vi "MDAQ_TestProgram.vi"() -> ()   [LabVIEW 2021]
uses:
  FunctionVIS/Status_Cluster.ctl
  FunctionVIS/CMD_ARG_Enum.ctl
  2434371f-5447-471b-b22c-6b5c2bc6bbb4.vi
panel:
  out "Delta4":dbl
  out "Delta 5":dbl
  out "Delta 3":dbl
  out "Delta 2":dbl
  out "Delta 1":dbl
  in  "stop":bool
  out "Intensity Graph":u32[][](graph)
  out "Test Ampl":T1(graph)
  in  "DeltaT":dbl
  in  "Freq":dbl
  in  "Bin":i32
  in  "VISA resource name":refnum<visa-resource-name>
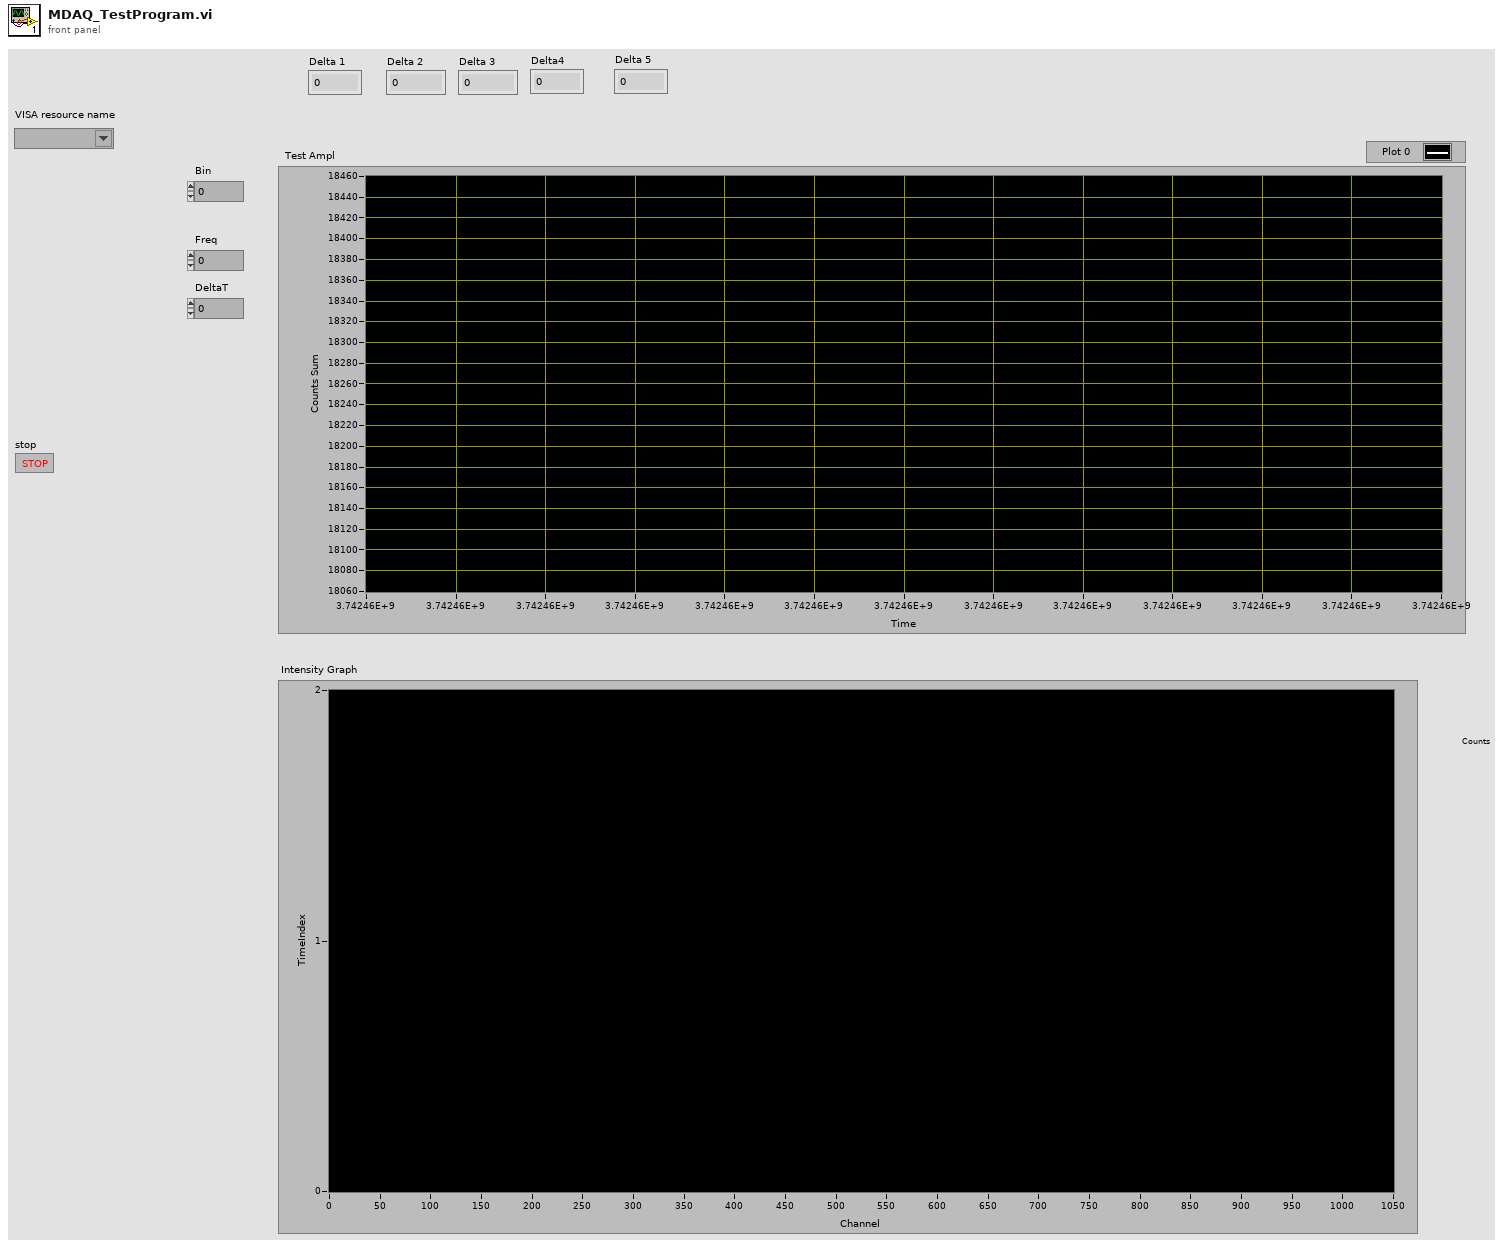
[diagram p1: front panel]
types:
  T1 = cluster{"seconds since 1Jan1904":timestamp, "sum":u32}[]
  T2 = typedef "Status_Cluster.ctl" = cluster{"CHAN":u32, "BASE":u32, "STEP":u32, "N_CYCLES":u32, "M_CYCLES":u32, "AMPLITUDE":u32, "GATESTRT":u32, "GATESTOP":u32, "Spectrum Array":u32[], "Spectrum Cycle":u32[][], "Cycle Timestamps":timestamp[], "Temperature Collect":dbl[]}
  T3 = typedef "CMD_ARG_Enum.ctl" = enum16{"N_Cycles", "GateStep", "ASCII_Spectrum", "Waveform", "GateStop", "GateStart", "Amplitude", "Frequency"}
  T4 = cluster{"seconds since 1Jan1904":timestamp, "sum":u32}
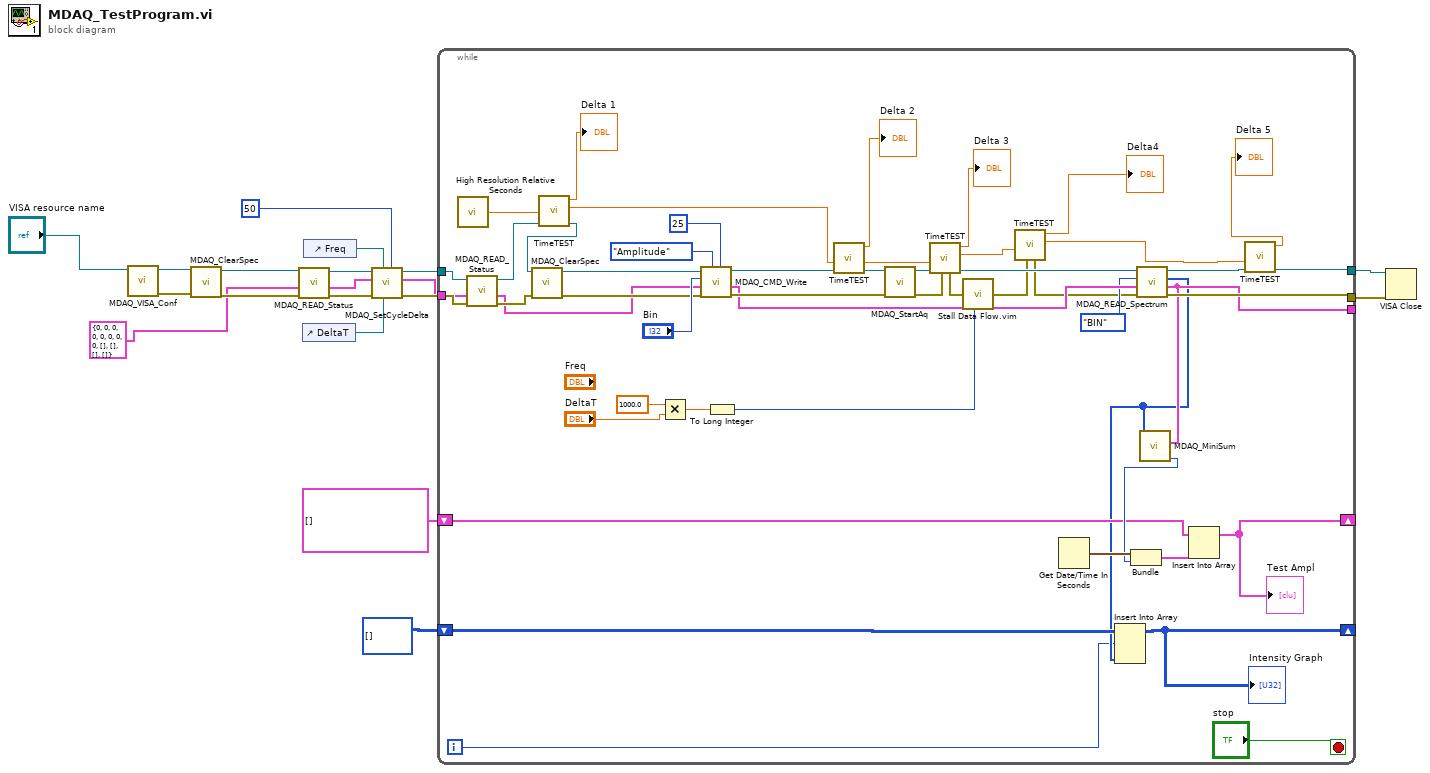
[diagram p0: block diagram]
diagram:
  n1 = call "MDAQ_VISA_Conf.vi"("VISA resource name"="VISA resource name") -> ("error out"=w17:errorcluster, "VISA resource name out"=w18:refnum<visa-resource-name>)  [unwired: 9 in]
  n2 = call "MDAQ_ClearSpec.vi"("error in (no error)"=w17, "VISA Refnum in"=w18) -> ("error out"=w6:errorcluster, "VISA Refnum out"=w7:refnum<visa-resource-name>)  [unwired: 8 in]
  n3 = call "MDAQ_READ_Status.vi"("error in"=w6, "Status_Cluster IN"=T2 {"CHAN"=0, "BASE"=0, "STEP"=0, "N_CYCLES"=0, "M_CYCLES"=0, "AMPLITUDE"=0, "GATESTRT"=0, "GATESTOP"=0, "Spectrum Array"=[], "Spectrum Cycle"=[], "Cycle Timestamps"=[], "Temperature Collect"=[]} ("Status_Cluster"), "VISA resource name"=w7) -> ("error out"=w8:errorcluster, "output cluster"=w4:T2, "VISA resource name out"=w9:refnum<visa-resource-name>)  [unwired: 6 in]
  n4 = control-ref of="DeltaT"() -> (w10:refnum<vi>)
  n5 = control-ref of="Freq"() -> (w3:refnum<vi>)
  n6 = call "MDAQ_SetCycleDelta.vi"("milliseconds to wait"=u32 50, "Delta T (s)"=w10, "Frequency"=w3, "error in"=w8, "Status_Cluster"=w4, "VISA resource name"=w9) -> ("error out"=w12:errorcluster, "Status_Cluster Out"=w1:T2, "VISA resource name out"=w11:refnum<visa-resource-name>)  [unwired: 3 in]
  n7 = while {
    tunnel: w11 -> [w21]
    tunnel: w12 -> [w25]
    tunnel: [w60] -> _
    shift-right: [w55] -> _
    shift-left: T1 [] -> [w56]
    tunnel: [w39] -> w16
    tunnel: [w61] -> w15
    shift-right: [w53] -> _
    shift-left: u32[][] [] -> [w54]
    tunnel: w1 -> [w23]
    i -> [w35]
    stop <- "stop" stop-if-true
    n8 = call <vilib>:"High Resolution Relative Seconds.vi"() -> ("relative seconds"=w50:dbl)
    n9 = call "MDAQ_READ_Status.vi"("error in"=w25, "Status_Cluster IN"=w23, "VISA resource name"=w21) -> ("error out"=w24:errorcluster, "output cluster"=w22:T2, "VISA resource name out"=w20:refnum<visa-resource-name>)  [unwired: 6 in]
    n10 = call "TimeTEST.vi"("VISA resource name"=w20, "relative seconds"=w50) -> ("VISA resource name 2"=w37:refnum<visa-resource-name>, "New Time"=w47:dbl, "Delta"=→"Delta 1":dbl)  [unwired: 6 in, 1 out]
    n11 = call "MDAQ_ClearSpec.vi"("error in (no error)"=w24, "VISA Refnum in"=w37) -> ("error out"=w38:errorcluster, "VISA Refnum out"=w36:refnum<visa-resource-name>)  [unwired: 8 in]
    n12 = Multiply(x=1000.0, y="DeltaT") -> (x*y=w64:dbl)
    n13 = call "MDAQ_CMD_Write.vi"("milliseconds to wait"=u32 25, "CMD"=CMD_ARG_Enum."Amplitude", "error in"=w38, "Status_Cluster"=w22, "ARG"="Bin", "VISA resource name"=w36) -> ("error out"=w68:errorcluster, "Status_Cluster Out"=w67:T2, "VISA resource name out"=w69:refnum<visa-resource-name>)  [unwired: 3 in]
    n14 = To Long Integer(number=w64) -> (32bit integer=w63:i32)
    n15 = call "TimeTEST.vi"("VISA resource name"=w69, "relative seconds"=w47) -> ("VISA resource name 2"=w48:refnum<visa-resource-name>, "New Time"=w44:dbl, "Delta"=→"Delta 2":dbl)  [unwired: 6 in, 1 out]
    n16 = call "MDAQ_StartAq.vi"("error in (no error)"=w68, "VISA Refnum in"=w48) -> ("error out"=w34:errorcluster, "VISA Refnum out"=w62:refnum<visa-resource-name>)  [unwired: 8 in]
    n17 = call "TimeTEST.vi"("error in (no error)"=w34, "VISA resource name"=w62, "relative seconds"=w44) -> ("VISA resource name 2"=w45:refnum<visa-resource-name>, "New Time"=w32:dbl, "Delta"=→"Delta 3":dbl, "error out"=w33:errorcluster)  [unwired: 5 in]
    n18 = call "Stall Data Flow.vim"("value in"=w33, "milliseconds to wait"=w63) -> ("value out"=w31:errorcluster)  [unwired: 1 out]
    n19 = call "TimeTEST.vi"("error in (no error)"=w31, "relative seconds"=w32) -> ("New Time"=w28:dbl, "Delta"=→"Delta4":dbl, "error out"=w30:errorcluster)  [unwired: 6 in, 1 out]
    n20 = Get Date/Time In Seconds() -> (seconds since 1Jan1904=w59:timestamp)
    n21 = call "MDAQ_READ_Spectrum.vi"("error in"=w30, "Status_Cluster IN"=w67, "Mode"=enum16{"BIN", "ASCII"}."BIN", "VISA resource name"=w45) -> ("error out"=w61:errorcluster, "output cluster"=w60:T2, "Output Array"=w52:u32[], "VISA resource name out"=w42:refnum<visa-resource-name>)  [unwired: 4 in]
    n22 = Insert Into Array(array=w54, index (row)=w35, new element=w52) -> (w53:u32[][])  [unwired: 1 in]
    "Intensity Graph" <- w53
    n23 = call "MDAQ_MiniSum.vi"("Status Cluster"=w60, "Spectrum"=w52) -> ("sum"=w58:u32)  [unwired: 9 in]
    n24 = Bundle("seconds since 1Jan1904"=w59, "sum"=w58) -> (w57:T4)  [unwired: 1 in]
    n25 = Insert Into Array(array=w56, new element=w57) -> (w55:T1)  [unwired: 1 in]
    "Test Ampl" <- w55
    n26 = call "TimeTEST.vi"("VISA resource name"=w42, "relative seconds"=w28) -> ("VISA resource name 2"=w39:refnum<visa-resource-name>, "Delta"=→"Delta 5":dbl)  [unwired: 6 in, 2 out]
  }
  n27 = VISA Close(VISA resource name=w16, error in (no error)=w15) -> ()  [unwired: 1 out]
